vi "Create_data_log_file_MHM.vi"(8 "error in (no error)":errorcluster, 10 "Export Folder Path":path, 11 "Byte Stream File in":refnum<file>) -> (0 "error out":errorcluster, 3 "Byte Stream File out":refnum<file>)   [LabVIEW 2013]
doc: "Creates a log file if not created already, only if reference is empty"
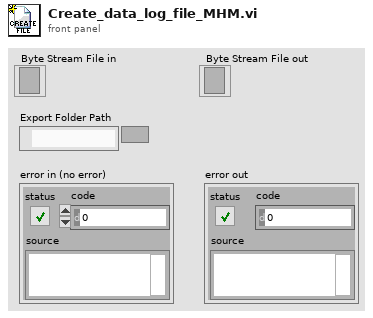
[diagram p1: front panel]
types:
  T1 = enum16{"open", "replace", "create", "open or create", "replace or create", "replace or create with confirmation"}
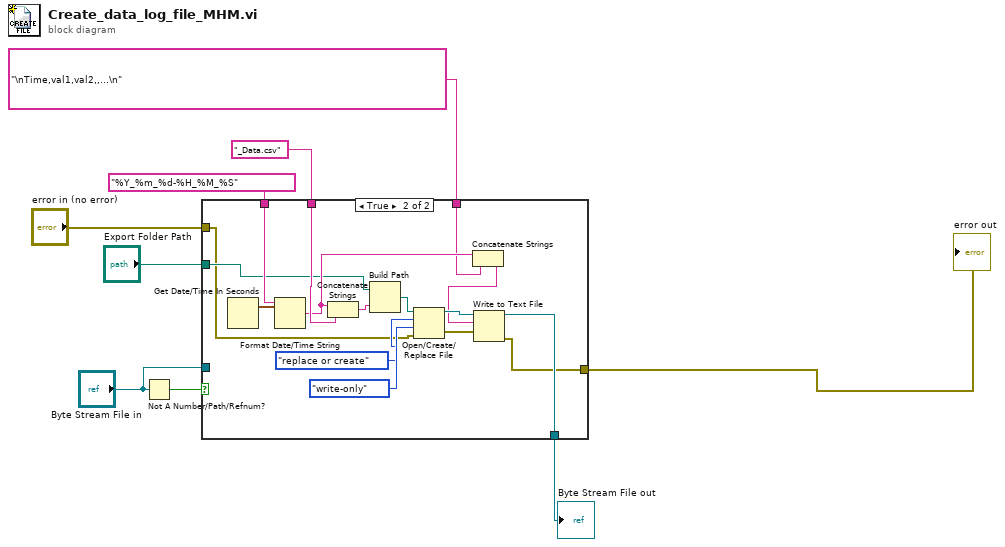
[diagram p0: block diagram]
diagram:
  n1 = Not A Number/Path/Refnum?(number/path/refnum="Byte Stream File in") -> (NaN/Path/Refnum?=w7:bool)
  n2 = case shown="True" w7 {
    tunnel: "_Data.csv" ("name or relative path") -> [_ w20]
    tunnel: "%Y_%m_%d-%H_%M_%S" -> [_ w19]
    tunnel: "Export Folder Path" -> [_ w16]
    tunnel: "error in (no error)" -> [w11 w15]
    tunnel: [w11 w13] -> w6
    tunnel: [w10 w14] -> w8
    tunnel: "Byte Stream File in" -> [w10 _]
    tunnel: "\nTime,val1,val2,,...\n" ("text") -> [_ w12]
    frame False {
      # "file alteady created, do not create another"
    }
    frame True {
      n3 = Get Date/Time In Seconds() -> (seconds since 1Jan1904=w27:timestamp)
      n4 = Format Date/Time String(time format string (%c)=w19, seconds (now)=w27) -> (date/time string=w17:string)  [unwired: 1 in]
      n5 = Concatenate Strings(w17, w20) -> (w21:string)
      n6 = Build Path(base path=w16, name or relative path=w21) -> (appended path=w23:path)
      n7 = Open/Create/Replace File(file path (use dialog)=w23, error in=w15, operation (0:open)=T1."replace or create", access (0:read/write)=enum16{"read/write", "read-only", "write-only"}."write-only") -> (refnum out=w22:refnum<file>, error out=w26:errorcluster)  [unwired: 2 in, 1 out]
      n8 = Concatenate Strings(w17, w12) -> (w18:string)
      n9 = Write to Text File(file (use dialog)=w22, text=w18, error in=w26) -> (refnum out=w14:refnum<file>, error out=w13:errorcluster)  [unwired: 1 in, 1 out]
    }
  }
  "Byte Stream File out" <- w8
  "error out" <- w6
